vi "Configure Source Output Characteristics.vi"(6 "Settling Mode (0: Smooth)":i32(ring) items=["Smooth", "Fast Range", "Fast Polarity", "Direct Current Range", "Smooth 100nA Range", "Fast All "], 7 "Enable Source Sink (F: Disable)":bool, 8 "error in (no error)":errorcluster, 9 "Output Action (0: No Action)":i32(ring) items=["No Action", "Turn Source Output Off"], 10 "Source Measure Unit Channel (0: Channel A)":i32(ring) items=["Channel A", "Channel B"], 11 "VISA resource name":refnum<visa-resource-name>) -> (0 "error out":errorcluster, 3 "VISA resource name out":refnum<visa-resource-name>)   [LabVIEW 2017, in "Keithley 2600 Series.lvlib"]
doc: "Configures the basic settings of the source output."
uses:
  <instrlib>/Keithley 2600 Series/Keithley 2600 Series.lvlib
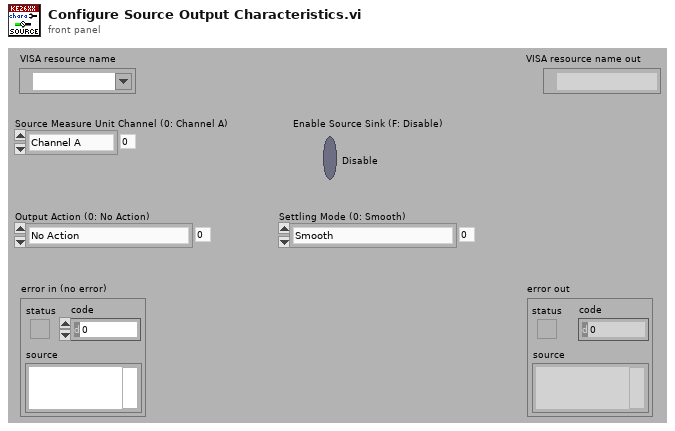
[diagram p1: front panel]
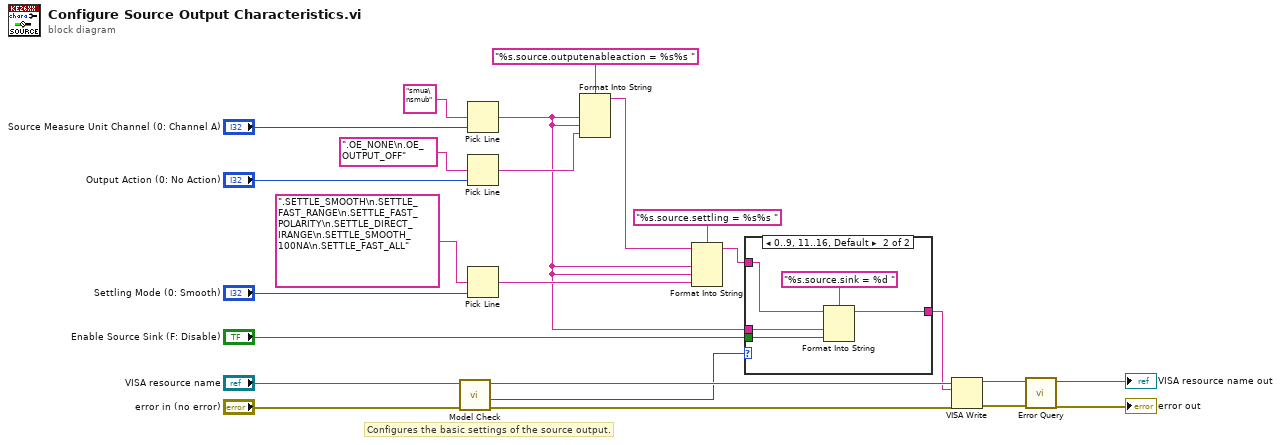
[diagram p0: block diagram]
diagram:
  # "Configures the basic settings of the source output."
  n1 = call <instrlib>:"Model Check.vi"("error in (no error)"="error in (no error)", "VISA resource name"="VISA resource name") -> ("error out"=w6:errorcluster, "Model"=w5:u16, "VISA resource name out"=w7:refnum<visa-resource-name>)  [unwired: 6 in, 1 out]
  n2 = Pick Line(multi-line string="smua\nsmub", line index="Source Measure Unit Channel (0: Channel A)") -> (output string=w10:string)  [unwired: 1 in]
  n3 = Pick Line(multi-line string=".OE_NONE\n.OE_OUTPUT_OFF", line index="Output Action (0: No Action)") -> (output string=w11:string)  [unwired: 1 in]
  n4 = Pick Line(multi-line string=".SETTLE_SMOOTH\n.SETTLE_FAST_RANGE\n.SETTLE_FAST_POLARITY\n.SETTLE_DIRECT_IRANGE\n.SETTLE_SMOOTH_100NA\n.SETTLE_FAST_ALL", line index="Settling Mode (0: Smooth)") -> (output string=w14:string)  [unwired: 1 in]
  n5 = Format Into String(format string="%s.source.outputenableaction = %s%s ", w10, w10, w11) -> (resulting string=w2:string)  [unwired: 2 in, 1 out]
  n6 = Format Into String(format string="%s.source.settling = %s%s ", initial string=w2, w10, w10, w14) -> (resulting string=w4:string)  [unwired: 1 in, 1 out]
  n7 = case shown="0..9, 11..16, Default" w5 {
    tunnel: w10 -> [_ w29]
    tunnel: w4 -> [w25 w28]
    tunnel: [w25 w27] -> w3
    tunnel: "Enable Source Sink (F: Disable)" -> [_ w26]
    frame 10 {
    }
    frame 0..9, 11..16, Default {
      n8 = Format Into String(format string="%s.source.sink = %d ", initial string=w28, w29, w26) -> (resulting string=w27:string)  [unwired: 1 in, 1 out]
    }
  }
  n9 = VISA Write(VISA resource name=w7, write buffer=w3, error in (no error)=w6) -> (VISA resource name out=w22:refnum<visa-resource-name>, error out=w21:errorcluster)  [unwired: 1 out]
  n10 = call <instrlib>:"Error Query.vi"("error in (no error)"=w21, "VISA resource name"=w22) -> ("error out"=→"error out":errorcluster, "VISA resource name out"=→"VISA resource name out":refnum<visa-resource-name>)  [unwired: 6 in, 2 out]
